vi "String to 1D Double Array.vi"(6 "Delimiter (,)":string=",", 8 "error in (no error)":errorcluster, 11 "String":string) -> (0 "error out":errorcluster, 3 "Array[]":dbl[](array[numeric]))   [LabVIEW 2014, in "SLL String.lvlib"]
uses:
  SLL String.lvlib
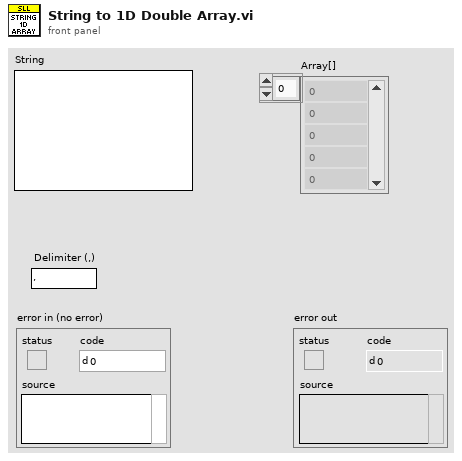
[diagram p1: front panel]
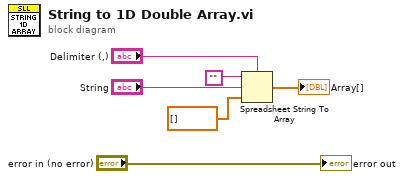
[diagram p0: block diagram]
diagram:
  n1 = Spreadsheet String To Array(delimiter (Tab)="Delimiter (,)", format string="", spreadsheet string="String", array type (2D Dbl)=dbl[] []) -> (array=→"Array[]":dbl[])
  "error out" <- "error in (no error)"
